vi "Send Trigger.vi"(8 "error in":errorcluster, 11 "4300 in":refnum<class "4300.lvclass">) -> (0 "error out":errorcluster, 3 "4300 out":refnum<class "4300.lvclass">)   [LabVIEW 2019, in "4300.lvlib" / "4300.lvclass"]
uses:
  Library/4300.lvclass
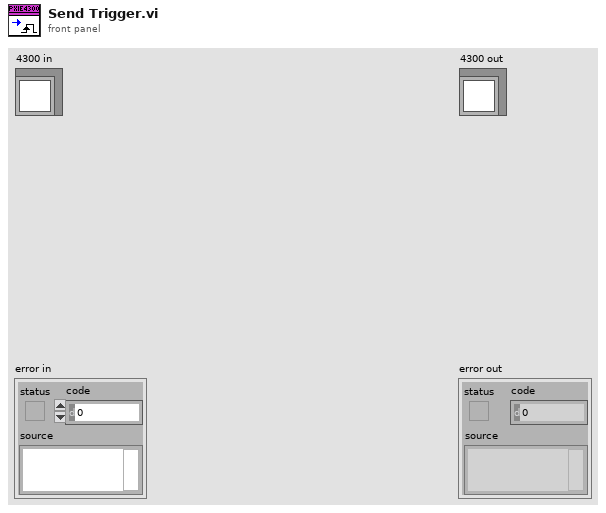
[diagram p1: front panel]
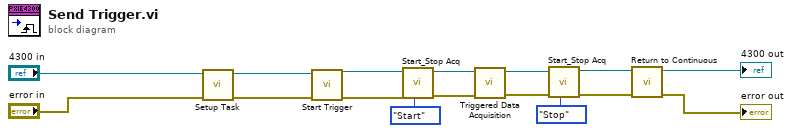
[diagram p0: block diagram]
diagram:
  n1 = call "Setup Task.vi"("error in"="error in", "4300 in"="4300 in") -> ("error out"=w1:errorcluster, "4300 out"=w2:refnum<class "4300.lvclass">)  [unwired: 8 in]
  n2 = call "Start Trigger.vi"("error in"=w1, "4300 in"=w2) -> ("error out"=w14:errorcluster, "4300 out"=w15:refnum<class "4300.lvclass">)  [unwired: 8 in]
  n3 = call-dynamic "Start_Stop Acq.vi"("Start/Stop"=enum16{"Start", "Stop"}."Start", "error in"=w14, "4300 in"=w15) -> ("error out"=w13:errorcluster, "4300 out"=w12:refnum<class "4300.lvclass">)  [unwired: 7 in]
  n4 = call "Triggered Data Acquisition.vi"("error in"=w13, "4300 in"=w12) -> ("error out"=w10:errorcluster, "4300 out"=w9:refnum<class "4300.lvclass">)  [unwired: 7 in, 1 out]
  n5 = call-dynamic "Start_Stop Acq.vi"("Start/Stop"=enum16{"Start", "Stop"}."Stop", "error in"=w10, "4300 in"=w9) -> ("error out"=w7:errorcluster, "4300 out"=w8:refnum<class "4300.lvclass">)  [unwired: 7 in]
  n6 = call "Return to Continuous.vi"("error in"=w7, "4300 in"=w8) -> ("error out"=→"error out":errorcluster, "4300 out"=→"4300 out":refnum<class "4300.lvclass">)  [unwired: 8 in]
